vi "Base Path Init.vi"(8 "error in":errorcluster, 11 "Folder name":string) -> (0 "error out":errorcluster, 3 "Folder Path":path)   [LabVIEW 2019]
doc: "Return path to folder inside project base directory. If folder does not exist - create it."
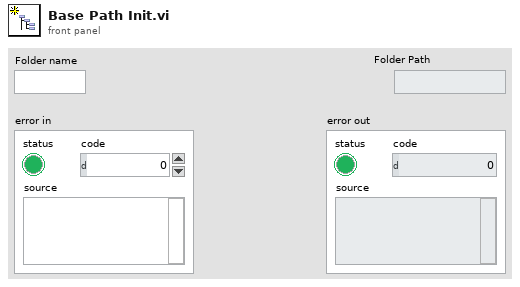
[diagram p1: front panel]
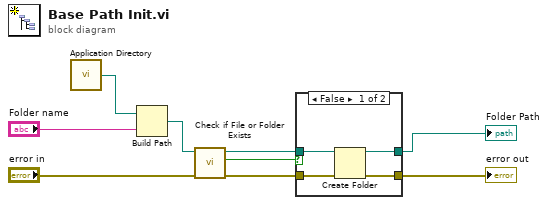
[diagram p0: block diagram]
diagram:
  n1 = call <vilib>:"Application Directory.vi"() -> ("Application Directory"=w5:path)
  n2 = Build Path(base path=w5, name or relative path="Folder name") -> (appended path=w9:path)
  n3 = call <vilib>:"Check if File or Folder Exists.vi"("error in (no error)"="error in", "path"=w9) -> ("error out"=w6:errorcluster, "file or folder exists?"=w8:bool, "dup path"=w7:path)  [unwired: 7 in]
  n4 = case shown="False" w8 {
    tunnel: w7 -> [w13 w15]
    tunnel: w6 -> [w12 w14]
    tunnel: [w10 w15] -> w2
    tunnel: [w11 w14] -> w3
    frame False {
      n5 = Create Folder(path (use dialog)=w13, error in=w12) -> (created path=w10:path, error out=w11:errorcluster)  [unwired: 1 in, 1 out]
    }
    frame True {
    }
  }
  "error out" <- w3
  "Folder Path" <- w2
